vi "Init.vi"(0 "VISA resource name":refnum<visa-resource-name>, 11 "error in (no error)":errorcluster) -> (4 "VISA resource name out":refnum<visa-resource-name>, 6 "Init Status":bool, 15 "error out":errorcluster)   [LabVIEW 2020]
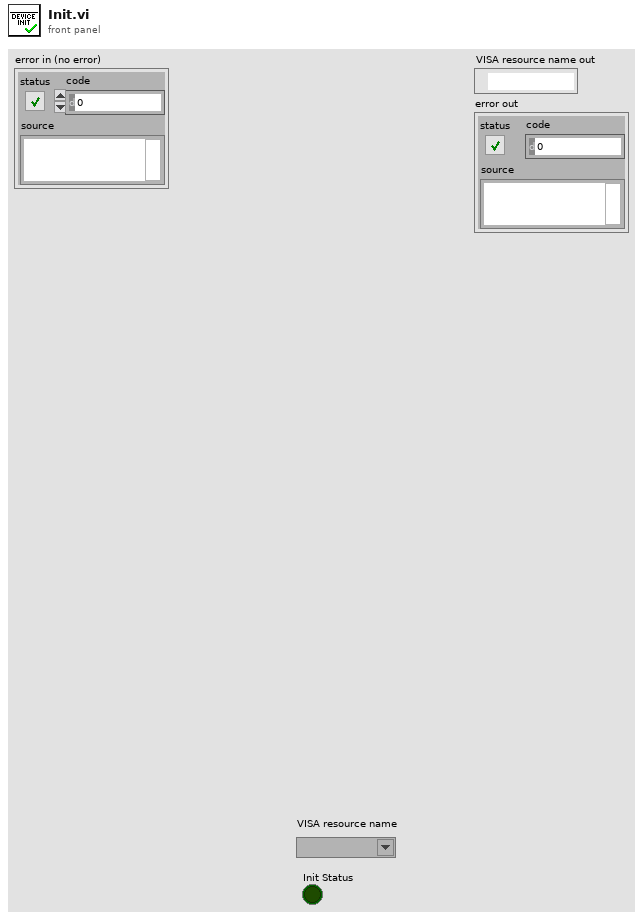
[diagram p1: front panel]
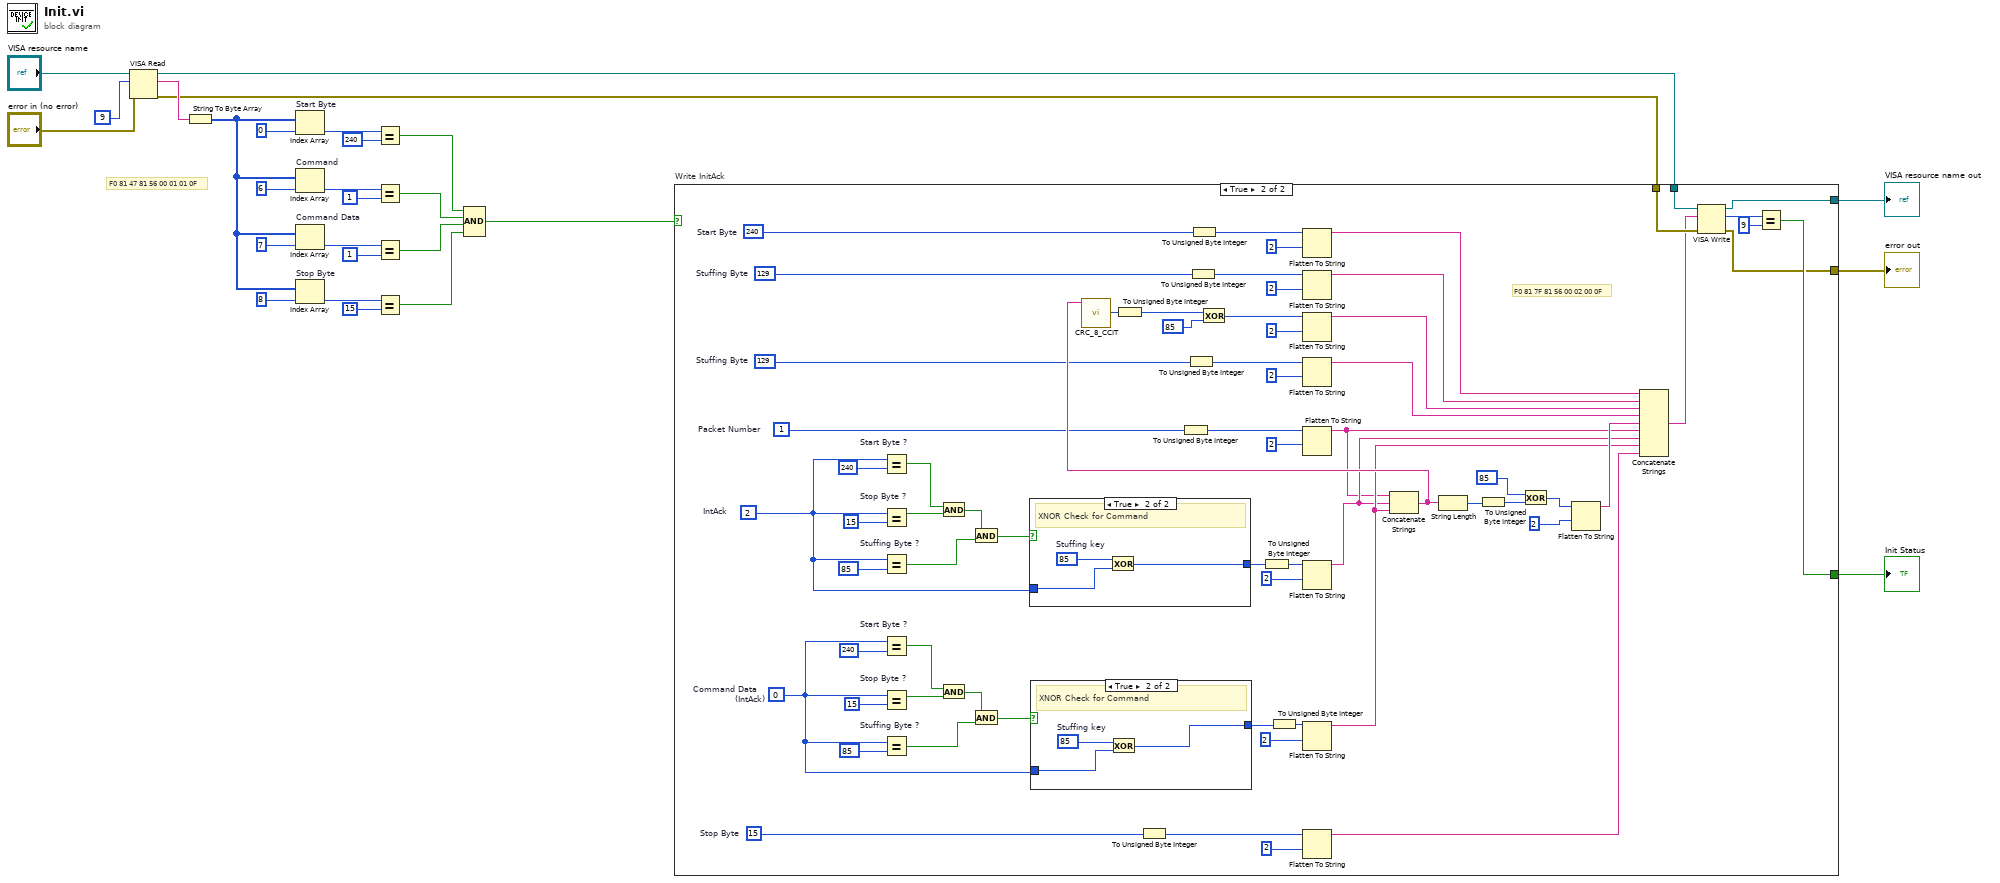
[diagram p0: block diagram]
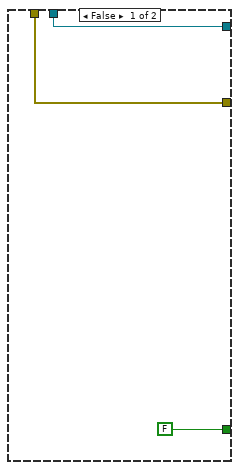
[diagram p2: hidden frame]
diagram:
  # "F0 81 47 81 56 00 01 01 0F"
  n1 = VISA Read(VISA resource name="VISA resource name", byte count=9 ("Bytes to Read"), error in (no error)="error in (no error)") -> (VISA resource name out=w7:refnum<visa-resource-name>, read buffer=w14:string, error out=w8:errorcluster)  [unwired: 1 out]
  n2 = String To Byte Array(string=w14) -> (unsigned byte array=w23:u8[])
  n3 = Index Array "Start Byte"(array=w23, index=0) -> (element=w21:u8)
  n4 = Index Array "Command"(array=w23, index=6) -> (element=w17:u8)
  n5 = Index Array "Command Data"(array=w23, index=7) -> (element=w16:u8)
  n6 = Index Array "Stop Byte"(array=w23, index=8) -> (element=w15:u8)
  n7 = Equal?(x=w21, y=u16 240) -> (x = y?=w12:bool)
  n8 = Equal?(x=w17, y=u16 1) -> (x = y?=w11:bool)
  n9 = Equal?(x=w16, y=u16 1) -> (x = y?=w10:bool)
  n10 = Equal?(x=w15, y=u16 15) -> (x = y?=w9:bool)
  n11 = Compound Arithmetic op=AND(w12, w11, w10, w9) -> (w4:bool)
  n12 = case "Write InitAck" shown="True" w4 {
    tunnel: w7 -> [w28 w39]
    tunnel: w8 -> [w29 w38]
    tunnel: [FALSE w34] -> w5
    tunnel: [w28 w32] -> w2
    tunnel: [w29 w31] -> w1
    frame False {
    }
    frame True {
      w37 = 1  # Packet Number
      w55 = 15  # Stop Byte
      w58 = 129  # Stuffing Byte
      w59 = 129  # Stuffing Byte
      w57 = 240  # Start Byte
      w78 = 0  # Command Data               (IntAck)
      w77 = 2  # IntAck
      # "F0 81 7F 81 56 00 02 00 0F"
      n13 = Equal? "Start Byte ?"(x=w77, y=240 ("IntAck")) -> (x = y?=w40:bool)
      n14 = Equal? "Stop Byte ?"(x=w77, y=15 ("IntAck")) -> (x = y?=w41:bool)
      n15 = Equal? "Stuffing Byte ?"(x=w77, y=85 ("IntAck")) -> (x = y?=w43:bool)
      n16 = Equal? "Start Byte ?"(x=w78, y=240 ("IntAck")) -> (x = y?=w45:bool)
      n17 = Equal? "Stop Byte ?"(x=w78, y=15 ("IntAck")) -> (x = y?=w46:bool)
      n18 = Equal? "Stuffing Byte ?"(x=w78, y=85 ("IntAck")) -> (x = y?=w48:bool)
      n19 = And(x=w40, y=w41) -> (x .and. y?=w42:bool)
      n20 = And(x=w45, y=w46) -> (x .and. y?=w47:bool)
      n21 = And(x=w42, y=w43) -> (x .and. y?=w44:bool)
      n22 = And(x=w47, y=w48) -> (x .and. y?=w49:bool)
      n23 = case shown="True" w44 {
        tunnel: w77 -> [w102 w105]
        tunnel: [w102 w103] -> w80
        frame False {
        }
        frame True {
          w104 = 85  # Stuffing key
          # "XNOR Check for Command"
          n24 = Exclusive Or(1:w105, 2:w104) -> (0:w103:i32)
        }
      }
      n25 = case shown="True" w49 {
        tunnel: w78 -> [w98 w101]
        tunnel: [w98 w99] -> w79
        frame False {
        }
        frame True {
          w100 = 85  # Stuffing key
          # "XNOR Check for Command"
          n26 = Exclusive Or(1:w101, 2:w100) -> (0:w99:i32)
        }
      }
      n27 = To Unsigned Byte Integer(number=w55) -> (unsigned 8bit integer=w56:u8)
      n28 = To Unsigned Byte Integer(number=w37) -> (unsigned 8bit integer=w89:u8)
      n29 = To Unsigned Byte Integer(number=w59) -> (unsigned 8bit integer=w62:u8)
      n30 = To Unsigned Byte Integer(number=w58) -> (unsigned 8bit integer=w61:u8)
      n31 = To Unsigned Byte Integer(number=w57) -> (unsigned 8bit integer=w60:u8)
      n32 = To Unsigned Byte Integer(number=w80) -> (unsigned 8bit integer=w88:u8)
      n33 = To Unsigned Byte Integer(number=w79) -> (unsigned 8bit integer=w87:u8)
      n34 = Flatten To String(anything=w60, byte order (0:big-endian, network order)=2) -> (data string=w50:string)  [unwired: 2 in, 2 out]
      n35 = Flatten To String(anything=w61, byte order (0:big-endian, network order)=2) -> (data string=w51:string)  [unwired: 2 in, 2 out]
      n36 = Flatten To String(anything=w62, byte order (0:big-endian, network order)=2) -> (data string=w53:string)  [unwired: 2 in, 2 out]
      n37 = Flatten To String(anything=w89, byte order (0:big-endian, network order)=2) -> (data string=w81:string)  [unwired: 2 in, 2 out]
      n38 = Flatten To String(anything=w88, byte order (0:big-endian, network order)=2) -> (data string=w82:string)  [unwired: 2 in, 2 out]
      n39 = Flatten To String(anything=w87, byte order (0:big-endian, network order)=2) -> (data string=w83:string)  [unwired: 2 in, 2 out]
      n40 = Flatten To String(anything=w56, byte order (0:big-endian, network order)=2) -> (data string=w54:string)  [unwired: 2 in, 2 out]
      n41 = Concatenate Strings(w81, w82, w83) -> (w91:string)
      n42 = call "CRC_8_CCIT.vi"("Data String"=w91) -> ("Numeric"=w90:u8)  [unwired: 10 in]
      n43 = To Unsigned Byte Integer(number=w90) -> (unsigned 8bit integer=w93:u8)
      n44 = Exclusive Or(1:u8 85, 2:w93) -> (0:w92:u8)
      n45 = Flatten To String(anything=w92, byte order (0:big-endian, network order)=2) -> (data string=w52:string)  [unwired: 2 in, 2 out]
      n46 = String Length(string=w91) -> (length=w85:i32)
      n47 = To Unsigned Byte Integer(number=w85) -> (unsigned 8bit integer=w96:u8)
      n48 = Exclusive Or(1:w96, 2:u8 85) -> (0:w95:u8)
      n49 = Flatten To String(anything=w95, byte order (0:big-endian, network order)=2) -> (data string=w86:string)  [unwired: 2 in, 2 out]
      n50 = Concatenate Strings(w50, w51, w52, w53, w86, w81, w82, w83, w54) -> (w33:string)
      n51 = VISA Write(VISA resource name=w39, write buffer=w33, error in (no error)=w38) -> (VISA resource name out=w32:refnum<visa-resource-name>, return count=w36:u32, error out=w31:errorcluster)
      n52 = Equal?(x=w36, y=9) -> (x = y?=w34:bool)
    }
  }
  "Init Status" <- w5
  "VISA resource name out" <- w2
  "error out" <- w1
